vi "RawAttrMap.vi"() -> (3 "Variant":variant)   [LabVIEW 2019, in "lv-apt-json-file.lvlib"]
uses:
  lv-apt-json-file.lvlib
  Def-AttrMap -- Map.ctl
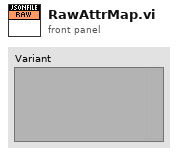
[diagram p1: front panel]
types:
  T1 = typedef "lv-apt-json-file.lvlib/Def-AttrMap -- Map.ctl" = map{string, string}
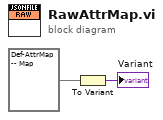
[diagram p0: block diagram]
diagram:
  n1 = To Variant(anything=T1 {}) -> (Variant=→"Variant":variant)
